vi "Thermometer.vi"(1 "Temp Scale":bool) -> (0 "Thermometer":dbl(slide) scale=0.0..100.0)   [LabVIEW 2025]
doc: "This VI measures temperature using the temperarture sensor on the DAQ Signal Accessory."
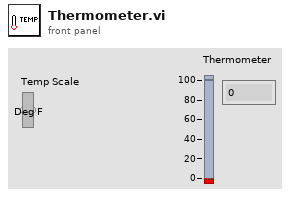
[diagram p1: front panel]
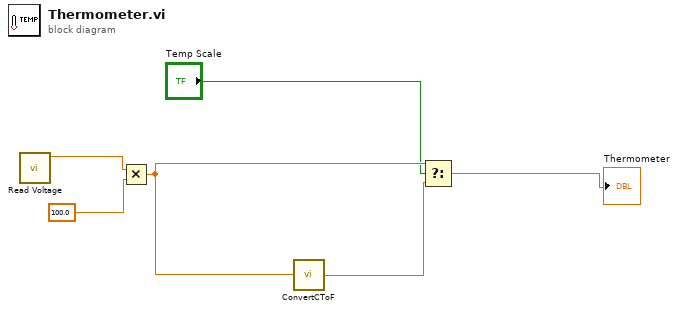
[diagram p0: block diagram]
diagram:
  n1 = call "Read Voltage.vi"() -> ("voltage"=w5:dbl)  [unwired: 6 in, 1 out]
  n2 = Multiply(x=w5, y=100.0) -> (x*y=w4:dbl)
  n3 = call "ConvertCToF.vi"("deg C"=w4) -> ("deg F"=w2:dbl)
  n4 = Select(t=w4, s="Temp Scale", f=w2) -> (s? t:f=→"Thermometer":dbl)
